vi "CSTR1.vi"(11 "Fuel Input":dbl) -> (3 "Reaction heat":dbl, 4 "CSTR Temp degC":dbl)   [LabVIEW 2020]
uses:
  <vilib>/Simulation/Implementation/Shared/SIMSCR Execution Mode.ctl
  <vilib>/Simulation/Scripting/Companion Diagram/SimConfigNode/SimParams.ctl
  <vilib>/Simulation/Scripting/Companion Diagram/SimConfigNode/_simSolvers.ctl
  <vilib>/Simulation/Param Hierarchy/Typedefs/SIMPH Param Control Actions.ctl
  <vilib>/Simulation/Implementation/Shared/NILVSim_ParamChanged.vi
  <vilib>/Simulation/Implementation/Shared/NILVSIM_BeginStep.vi
  <vilib>/Simulation/Utility/Implementation/NILVSim Memory.llb/NILVSim Memory (core).vi
  <vilib>/Simulation/ContinuousLinear/Implementation/NILVSim Transfer Function.llb/SIM Transfer Function Distributor (SISO).vi
  <vilib>/Simulation/ContinuousLinear/Implementation/NILVSim Transfer Function.llb/SIM Transfer Function Collector (SISO).vi
  <vilib>/Simulation/Implementation/Shared/NILVSim_Manager.vi
  <vilib>/Utility/error.llb/Clear Errors.vi
  <vilib>/Simulation/Implementation/Shared/NILVSim_FinalizeModel.vi
  <vilib>/Simulation/Implementation/Shared/SIM Unbundle Sim Info.vi
  <vilib>/Simulation/Implementation/Shared/NILVSim_Initialize.vi
  <vilib>/Simulation/Utility/Implementation/NILVSim Get Time and IsAcceptedStep.vi
  <vilib>/Simulation/Implementation/Shared/NILVSim_GetModelError.vi
  <vilib>/Simulation/Implementation/Shared/SIM SimErrorHandler.vi
  <vilib>/Simulation/Implementation/Shared/SIMSH Read Queue.vi
  <vilib>/Simulation/Implementation/Shared/SIM Bundle Sim Info.vi
  <vilib>/Simulation/Scripting/Companion Diagram/SimConfigNode/SimDog.xnode
  <vilib>/Simulation/ContinuousLinear/Implementation/NILVSim Transfer Function.llb/SIM Transfer Function (SISO).vi
  <vilib>/Simulation/Implementation/XNodeFramework/SimXNode/SimX.xnode
  <vilib>/Simulation/Implementation/Shared/NI_SIM_Implementation.lvlib
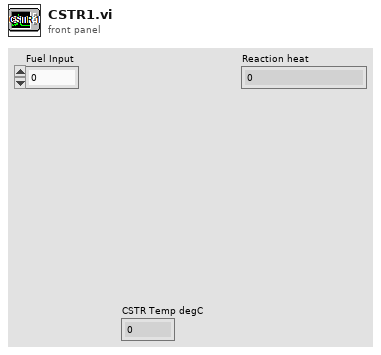
[diagram p1: front panel]
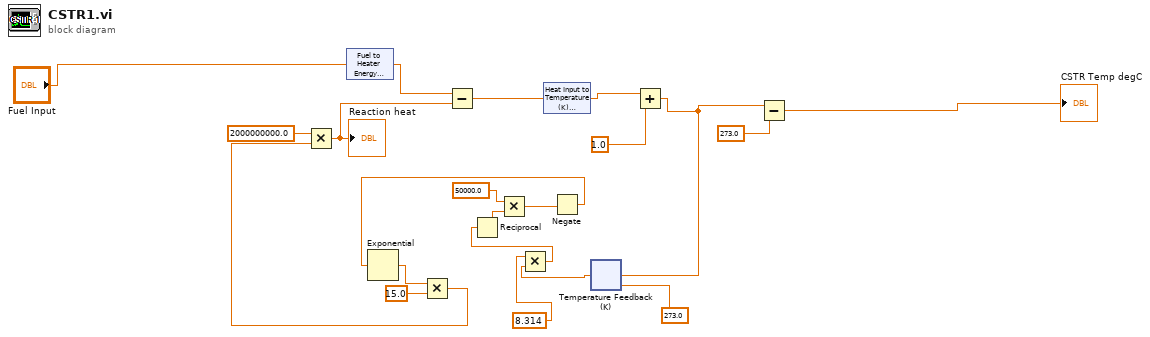
[diagram p0: block diagram]
diagram:
  n1 = xnode "Fuel to Heater Energy\nTransfer Fn"("input u(t)"="Fuel Input") -> ("output y(t)"=w19:dbl)  [unwired: 3 in, 1 out]
  n2 = Multiply ("Multiply 4")(x=2000000000.0, y=w12) -> (x*y=w15:dbl)
  "Reaction heat" <- w15
  n3 = Subtract ("Subtract 2")(x=w19, y=w15) -> (x-y=w14:dbl)
  n4 = xnode "Heat Input to Temperature (K)\nTransfer Function"("input u(t)"=w14) -> ("output y(t)"=w16:dbl)  [unwired: 3 in, 1 out]
  n5 = Add(x=w16, y=1.0 ("y 3")) -> (x+y=w18:dbl)
  n6 = xnode "Temperature Feedback\n(K)"("input"=w18, "initial value"=273.0) -> ("output"=w3:dbl)  [unwired: 4 in]
  n7 = Multiply(x=8.314 ("Constant"), y=w3) -> (x*y=w5:dbl)
  n8 = Reciprocal(x=w5) -> (1/x=w7:dbl)
  n9 = Multiply ("Multiply 2")(x=50000.0 ("Constant 2"), y=w7) -> (x*y=w8:dbl)
  n10 = Negate(x=w8) -> (-x=w9:dbl)
  n11 = Exponential(1:w9) -> (0:w10:dbl)
  n12 = Multiply ("Multiply 3")(x=w10, y=15.0 ("y 2")) -> (x*y=w12:dbl)
  n13 = Subtract(x=w18, y=273.0) -> (x-y=→"CSTR Temp degC":dbl)
